vi "Calculate Shortest Distance.vi"(10 "Target":dbl, 11 "Robot Heading":dbl) -> (2 "Shortest Distance":dbl)   [LabVIEW 2015]
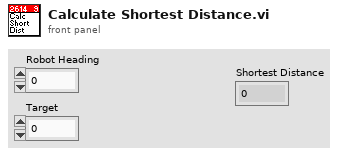
[diagram p1: front panel]
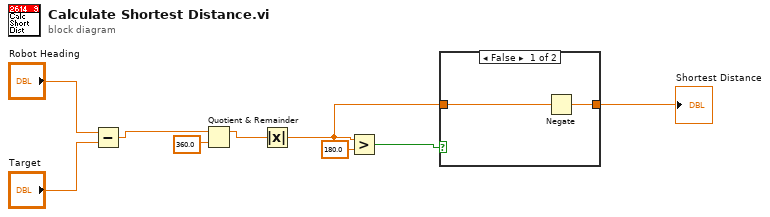
[diagram p0: block diagram]
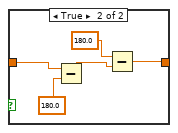
[diagram p2: hidden frame]
diagram:
  n1 = Subtract(x="Robot Heading", y="Target") -> (x-y=w4:dbl)
  n2 = Quotient & Remainder(x=w4, y=360.0) -> (x-y*floor(x/y)=w3:dbl)  [unwired: 1 out]
  n3 = Absolute Value(x=w3) -> (abs(x)=w6:dbl)
  n4 = Greater?(x=w6, y=180.0) -> (0:w7:bool)
  n5 = case shown="False" w7 {
    tunnel: w6 -> [w11 w13]
    tunnel: [w10 w16] -> w5
    frame False {
      n6 = Negate(x=w11) -> (-x=w10:dbl)
    }
    frame True {
      n7 = Subtract(x=w13, y=180.0 ("x")) -> (x-y=w14:dbl)
      n8 = Subtract(x=180.0, y=w14) -> (x-y=w16:dbl)
    }
  }
  "Shortest Distance" <- w5
